vi "Main.vi"() -> ()   [LabVIEW 2021]
doc: "The myRIO Project template acquires acceleration data from the onboard accelerometer and displays the changes of acceleration values in a waveform chart."
uses:
  <vilib>/Platform/TimedLoop/XDataNode/timing_clust.ctl
  <vilib>/Platform/TimedLoop/XDataNode/nitl_modes.ctl
  <vilib>/Platform/TimedLoop/XDataNode/wakeup.ctl
  <vilib>/myRIO/Instrument Drivers/Onboard IO/I2C/typedefs/I2C User Configuration.ctl
  <vilib>/myRIO/Instrument Drivers/Onboard IO/I2C/typedefs/I2C Transfer Rate.ctl
  <vilib>/myRIO/Instrument Drivers/Onboard IO/I2C/typedefs/I2C Reference.ctl
  <vilib>/myRIO/Common/Instrument Driver Framework/Utilities/typedefs/myRIO Generic Hardware Reference.ctl
  <vilib>/myRIO/Common/Instrument Driver Framework/Utilities/typedefs/Hardware Version Enum.ctl
  <vilib>/myRIO/Common/Instrument Driver Framework/Utilities/typedefs/myRIO v1.0 Reference.ctl
  <vilib>/myRIO/Common/Instrument Driver Framework/Utilities/typedefs/Generic FPGA Reference.ctl
  <vilib>/myRIO/Common/Instrument Driver Framework/myRIO v1.0/I2C/typedefs/I2C Channels Enum.ctl
  <vilib>/myRIO/Instrument Drivers/Onboard IO/I2C/typedefs/I2C Configuration.ctl
  <vilib>/userDefined/High Color/nirio_resource_hc.ctl
  <vilib>/myRIO/Instrument Drivers/Onboard IO/UART/typedef/VISA Configuration.ctl
  <vilib>/myRIO/Instrument Drivers/Onboard IO/DIO/typedefs/DIO Reference.ctl
  <vilib>/myRIO/Common/Instrument Driver Framework/myRIO v1.0/DIO/typedefs/DIO Channels List.ctl
  <vilib>/myRIO/Common/Instrument Driver Framework/myRIO v1.0/DIO/typedefs/DIO Channels Enum.ctl
  <vilib>/myRIO/Instrument Drivers/Onboard IO/PWM/typedefs/PWM Reference.ctl
  <vilib>/myRIO/Common/Instrument Driver Framework/myRIO v1.0/PWM/typedefs/PWM Channels Enum.ctl
  <vilib>/myRIO/Instrument Drivers/Onboard IO/PWM/typedefs/PWM Configuration.ctl
  <vilib>/myRIO/Common/Instrument Driver Framework/Utilities/vis/Is FPGA Ref Available.vi
  <vilib>/myRIO/Common/Instrument Driver Framework/myRIO v1.0/I2C/vis/myRIO v1.1 Open I2C.vi
  <vilib>/myRIO/Instrument Drivers/Onboard IO/I2C/vis/Configure.vi
  <vilib>/myRIO/Instrument Drivers/Onboard IO/I2C/vis/Write.vi
  <vilib>/myRIO/Instrument Drivers/Onboard IO/I2C/vis/Read.vi
  5875c5f5-a436-469e-884c-53e7f58b3f13.vi
  <vilib>/myRIO/Common/Instrument Driver Framework/myRIO v1.0/DIO/vis/myRIO v1.1 Open DIO.vi
  <vilib>/myRIO/Instrument Drivers/Onboard IO/DIO/vis/Write.vi
  6fa42901-1153-49b1-957e-1088346b90ec.vi
  <vilib>/myRIO/Common/Instrument Driver Framework/myRIO v1.0/PWM/vis/myRIO v1.1 Open PWM.vi
  <vilib>/myRIO/Instrument Drivers/Onboard IO/PWM/vis/Set Duty Cycle and Frequency.vi
  <vilib>/myRIO/Instrument Drivers/Onboard IO/I2C/vis/Write Read.vi
  <vilib>/myRIO/Common/Instrument Driver Framework/Utilities/vis/Validate Channels.vi
  <vilib>/myRIO/Common/Instrument Driver Framework/myRIO v1.0/I2C/vis/myRIO v1.0 Reserve I2C.vi
  <vilib>/myRIO/Common/Instrument Driver Framework/myRIO v1.0/DIO/vis/myRIO v1.0 Reserve DIO.vi
  <vilib>/myRIO/Common/Instrument Driver Framework/myRIO v1.0/PWM/vis/myRIO v1.0 Reserve PWM.vi
  <vilib>/myRIO/Common/Instrument Driver Framework/myRIO v1.0/I2C/vis/myRIO v1.0 Build MUX Configuration I2C.vi
  <vilib>/myRIO/Common/Instrument Driver Framework/myRIO v1.0/Resource Manager/vis/myRIO v1.0 Reserve Channel List.vi
  <vilib>/myRIO/Common/Instrument Driver Framework/myRIO v1.0/DIO/vis/myRIO v1.0 Build MUX Configuration DIO.vi
  <vilib>/myRIO/Common/Instrument Driver Framework/myRIO v1.0/PWM/vis/myRIO v1.0 Build MUX Configuration PWM.vi
  <vilib>/myRIO/Common/Instrument Driver Framework/myRIO v1.0/Resource Manager/vis/myRIO v1.0 Create Configuration List.vi
  <vilib>/myRIO/Common/Instrument Driver Framework/myRIO v1.0/Resource Manager/vis/myRIO v1.0 Reserve Channel.vi
  <vilib>/myRIO/Common/Instrument Driver Framework/myRIO v1.0/Resource Manager/vis/myRIO v1.0 Unreserve Channel.vi
  <vilib>/myRIO/Common/Instrument Driver Framework/myRIO v1.0/Resource Manager/vis/myRIO v1.0 Build Mutex Name.vi
  <vilib>/Utility/VariantDataType/GetNumericInfo.vi
  <vilib>/Utility/error.llb/Error Cluster From Error Code.vi
  <vilib>/myRIO/Common/Instrument Driver Framework/myRIO v1.0/myRIO v1.1 Open.vi
  <vilib>/myRIO/Common/Instrument Driver Framework/Utilities/vis/IO Manager.vi
  <vilib>/myRIO/Common/Instrument Driver Framework/Utilities/vis/Configuration Manager.vi
  <vilib>/myRIO/Common/Instrument Driver Framework/myRIO v1.0/Resource Manager/vis/myRIO v1.0 Configure IO.vi
  <vilib>/myRIO/Common/Instrument Driver Framework/myRIO v1.0/myRIO v1.0 Close.vi
  <vilib>/myRIO/Common/Instrument Driver Framework/myRIO v1.0/I2C/vis/myRIO v1.0 Configure I2C.vi
  <vilib>/myRIO/Common/Instrument Driver Framework/myRIO v1.0/I2C/vis/myRIO v1.0 Write I2C.vi
  <vilib>/myRIO/Common/Instrument Driver Framework/myRIO v1.0/I2C/vis/myRIO v1.0 Read I2C.vi
  <vilib>/myRIO/Common/Instrument Driver Framework/myRIO v1.0/DIO/vis/myRIO v1.0 Write DIO.vi
  <vilib>/Instr/_visa.llb/VISA Configure Serial Port (Instr).vi
  <vilib>/myRIO/Common/Instrument Driver Framework/myRIO v1.0/PWM/vis/myRIO v1.0 Write PWM.vi
  <vilib>/myRIO/Express VI/Onboard IO/I2C/I2C Express VI.xnode
  <vilib>/myRIO/Instrument Drivers/Onboard IO/I2C/vis/myRIO I2C Open.xnode
  <vilib>/platform/TimedLoop/XDataNode/XDataNode.xnode
  <vilib>/myRIO/Express VI/Onboard IO/DO/DO Express VI.xnode
  <vilib>/myRIO/Instrument Drivers/Onboard IO/DIO/vis/myRIO DIO Open.xnode
  <vilib>/myRIO/Express VI/Onboard IO/UART/UART Express VI.xnode
  <vilib>/myRIO/Express VI/Onboard IO/PWM/PWM Express VI.xnode
  <vilib>/myRIO/Instrument Drivers/Onboard IO/PWM/vis/myRIO PWM Open.xnode
  <vilib>/myRIO/Instrument Drivers/Onboard IO/I2C/I2C.lvlib
  <vilib>/Platform/TimedLoop/XDataNode/XDNodeRunTimeDep.lvlib
  <vilib>/myRIO/Instrument Drivers/Onboard IO/UART/UART.lvlib
  <vilib>/myRIO/Instrument Drivers/Onboard IO/DIO/DIO.lvlib
  <vilib>/myRIO/Instrument Drivers/Onboard IO/PWM/PWM.lvlib
panel:
  in  "Set Prox.\nAlert [in]":i32=5
  out "Distance to Tree [in]":dbl(slide) scale=6.0..60.0
  out "Thermometer [C]":dbl(slide) scale=0.0..30.0
  in  "Set Low Temp\nAlert [Celsius]":dbl=-1.0 format="%#_13g"
  out "Error":errorcluster
  out "# of Tree Alerts":i16
  out "# of Cold\nAlerts":i16
  out "MAXSONAR out":string
  out "Temperature [Celsius]":dbl
  out "Tree Proximity [in]":i32
  out "XY Graph":cluster{i32[], i32[]}[](graph)
  in  "stop":bool
  in  "Reset To Cabin":bool
  out "CMPS2 Bytes Read":u8[](array[numeric])
  out "X Y Gauss":dbl[](array[numeric])
  out "CMPS2 Status Register":bool[](array[boolean])
  out "ACL INT SOURCE":bool[](array[boolean])
  out "ACL Bytes Read":u8[](array[numeric])
  out "X ACL":i16 format="%.1f"
  out "Y ACL":i16 format="%.1f"
  out "Z ACL":i16 format="%.1f"
  out "Acceleration":i16
  out "Walking":bool
  out "Compass Case":u32
  out "Compass\nHeading":string="E"
  # "CABIN"
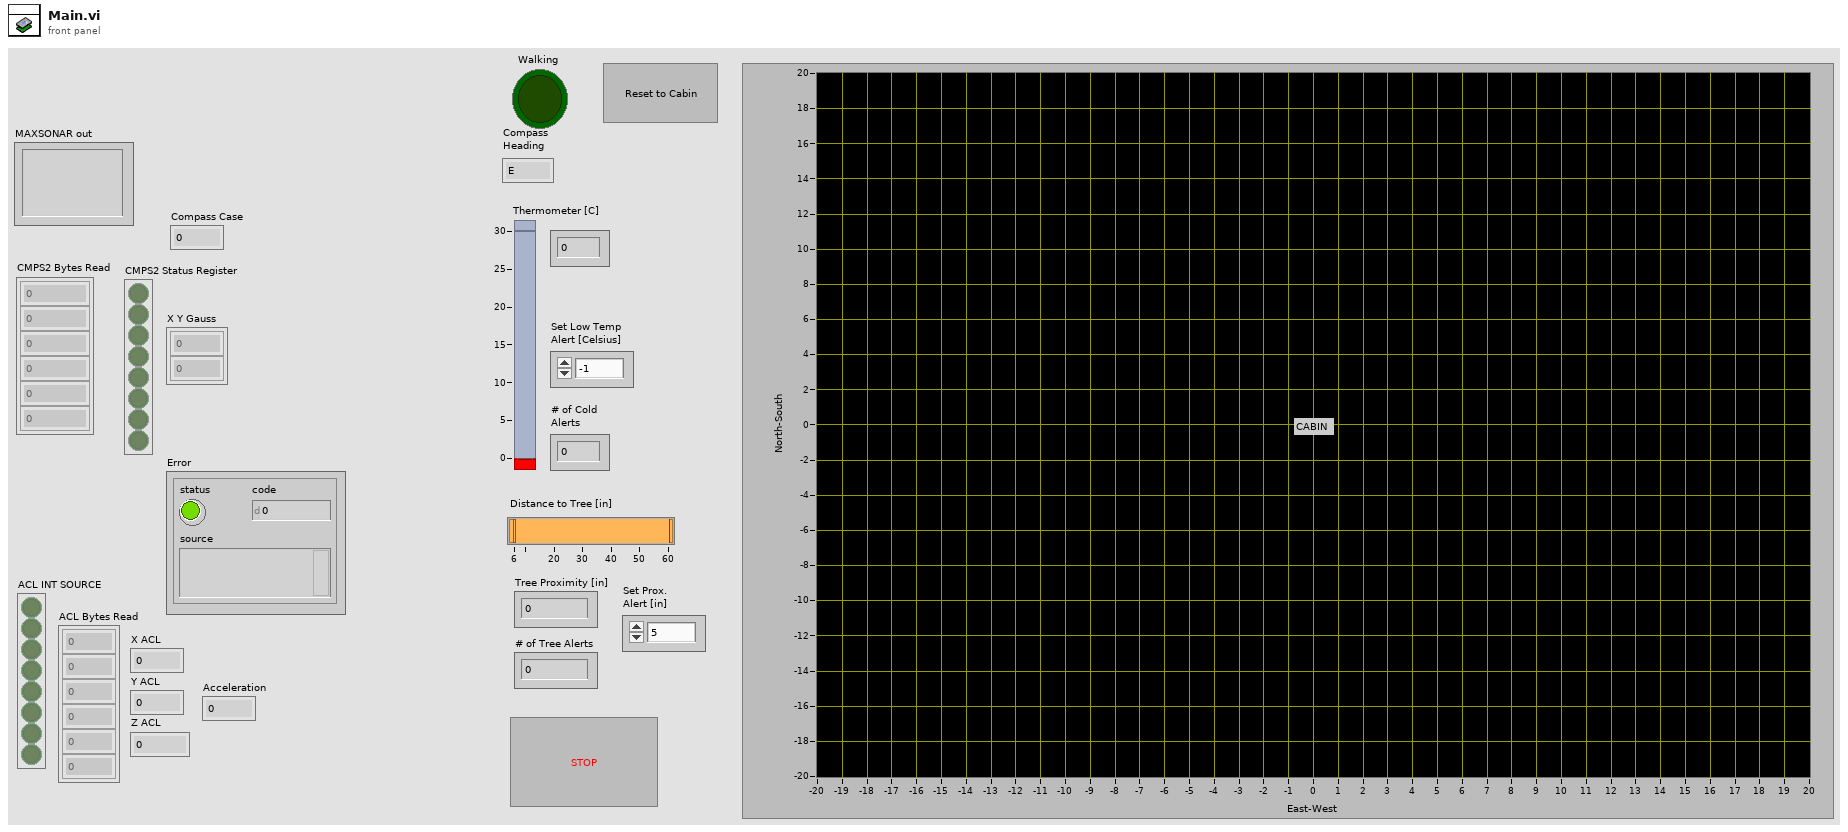
[diagram p1: front panel]
types:
  T1 = typedef "I2C.lvlib/I2C Reference.ctl" = cluster{"myRIO Reference":T2, "I2C Channels Enum":T6, "I2C Configuration":T7}
  T2 = typedef "myRIO Generic Hardware Reference.ctl" = cluster{"myRIO Model":T3, "myRIO Hardware Reference":T4}
  T3 = typedef "Hardware Version Enum.ctl" = enum16{"Unknown", "myRIO-1900", "myRIO-1950", "roboRIO", "NI ELVIS RIO CM", "ELVIS III"}
  T4 = typedef "myRIO v1.0 Reference.ctl" = cluster{"Generic FPGA Reference":T5, "Allow multiple opens":bool}
  T5 = typedef "Generic FPGA Reference.ctl" = refnum<k20>
  T6 = typedef "I2C Channels Enum.ctl" = enum16{"Not Connected", "A/I2C", "B/I2C", "I2C/I2C"}
  T7 = typedef "I2C.lvlib/I2C Configuration.ctl" = cluster{"I2C Transfer Rate":T8}
  T8 = typedef "I2C.lvlib/I2C Transfer Rate.ctl" = enum16{"Standard mode (100 kbps)", "Fast mode (400 kbps)"}
  T9 = typedef "I2C.lvlib/I2C User Configuration.ctl" = cluster{"I2C Transfer Rate":T8}
  T10 = typedef "nirio_resource_hc.ctl" = tag
  T11 = typedef "XDNodeRunTimeDep.lvlib/timing_clust.ctl" = cluster{"Expected End [f-1]":u64, "Actual End [f-1]":u64, "Finished Late? [f-1]":bool, "Expected End [i-1]":u64, "Actual End [i-1]":u64, "Finished Late? [i-1]":bool, "Expected Start [i]":u64, "Actual Start [i]":u64, "Expected Start [f]":u64, "Actual Start [f]":u64, "Source Name":string, "Structure Name":string, "Period":i64, "Deadline":i64, "Offset":i64, "Start":i64, "Priority":i32, "Timeout":i32, "Mode":T12, "Wakeup Reason":T13, "Error":errorcluster, "Source Type":string, "Secondary Source Type":string, "Global End Time":u64, "Global Start Time":u64, "Frame Duration":u64, "Iteration Duration":u64, "Assigned CPU":i32, "I/O Scan Engine Mode":u32}
  T12 = typedef "XDNodeRunTimeDep.lvlib/nitl_modes.ctl" = enum32{"No Change", "Process missed periods, maintain original phase", "Discard missed periods, maintain original phase", "Process missed periods, ignore original phase", "Discard missed periods, ignore original phase"}
  T13 = typedef "XDNodeRunTimeDep.lvlib/wakeup.ctl" = enum32{"Normal", "Aborted", "Asynchronous wakeup", "Timing source error", "Timed loop error", "Timeout"}
  T14 = typedef "PWM.lvlib/PWM Reference.ctl" = cluster{"myRIO Reference":T2, "PWM Channels Enum":T15, "PWM Configuration":T16}
  T15 = typedef "PWM Channels Enum.ctl" = enum16{"Not Connected", "C/PWM0", "C/PWM1", "A/PWM0", "A/PWM1", "A/PWM2", "A/PWM3", "A/PWM4", "A/PWM5", "A/PWM6", "A/PWM7", "A/PWM8", "A/PWM9", "A/PWM10", "A/PWM11", "A/PWM12", "A/PWM13", "A/PWM14", "A/PWM15", "A/PWM16", "A/PWM17", "A/PWM18", "A/PWM19", "B/PWM0", "B/PWM1", "B/PWM2", "B/PWM3", "B/PWM4", "B/PWM5", "B/PWM6", "B/PWM7", "B/PWM8", "B/PWM9", "B/PWM10", "B/PWM11", "B/PWM12", "B/PWM13", "B/PWM14", "B/PWM15", "B/PWM16", "B/PWM17", "B/PWM18", "B/PWM19", "PWM/PWM0", "PWM/PWM1", "PWM/PWM2", "PWM/PWM3", "PWM/PWM4", "PWM/PWM5", "PWM/PWM6", "PWM/PWM7", "PWM/PWM8", "PWM/PWM9"}
  T16 = typedef "PWM.lvlib/PWM Configuration.ctl" = cluster{"Frequency":dbl, "Duty Cycle":dbl}
  T17 = typedef "DIO.lvlib/DIO Reference.ctl" = cluster{"myRIO Reference":T2, "DIO Channels List":T18}
  T18 = typedef "DIO Channels List.ctl" = T19[]
  T19 = typedef "DIO Channels Enum.ctl" = enum16{"Not Connected", "C/DIO0", "C/DIO1", "C/DIO2", "C/DIO3", "C/DIO4", "C/DIO5", "C/DIO6", "C/DIO7", "A/DIO0", "A/DIO1", "A/DIO2", "A/DIO3", "A/DIO4", "A/DIO5", "A/DIO6", "A/DIO7", "A/DIO8", "A/DIO9", "A/DIO10", "A/DIO11", "A/DIO12", "A/DIO13", "A/DIO14", "A/DIO15", "A/DIO16", "A/DIO17", "A/DIO18", "A/DIO19", "B/DIO0", "B/DIO1", "B/DIO2", "B/DIO3", "B/DIO4", "B/DIO5", "B/DIO6", "B/DIO7", "B/DIO8", "B/DIO9", "B/DIO10", "B/DIO11", "B/DIO12", "B/DIO13", "B/DIO14", "B/DIO15", "B/DIO16", "B/DIO17", "B/DIO18", "B/DIO19", "LED0", "LED1", "LED2", "LED3", "Button0", "DIO/DIO0", "DIO/DIO1", "DIO/DIO2", "DIO/DIO3", "DIO/DIO4", "DIO/DIO5", "DIO/DIO6", "DIO/DIO7", "DIO/DIO8", "DIO/DIO9", "SPI/CS0", "SPI/CS1", "SPI/CS2", "SPI/CS3", "LED RADIO (Green)", "LED RADIO (Red)", "LED COMM (Green)", "LED COMM (Red)", "LED MODE (Green)", "LED MODE (Red)"}
  T20 = typedef "UART.lvlib/VISA Configuration.ctl" = cluster{"baud rate (9600)":u32, "data bits (8)":u16, "parity (0:none)":enum16{"None", "Odd", "Even", "Mark", "Space"}, "stop bits (10: 1 bit)":u16, "flow control (0:none)":u16, "termination char\n(0xA = '\\n' = LF) ":u8, "Enable Termination\nChar (T)":bool, "timeout (10sec)":u32}
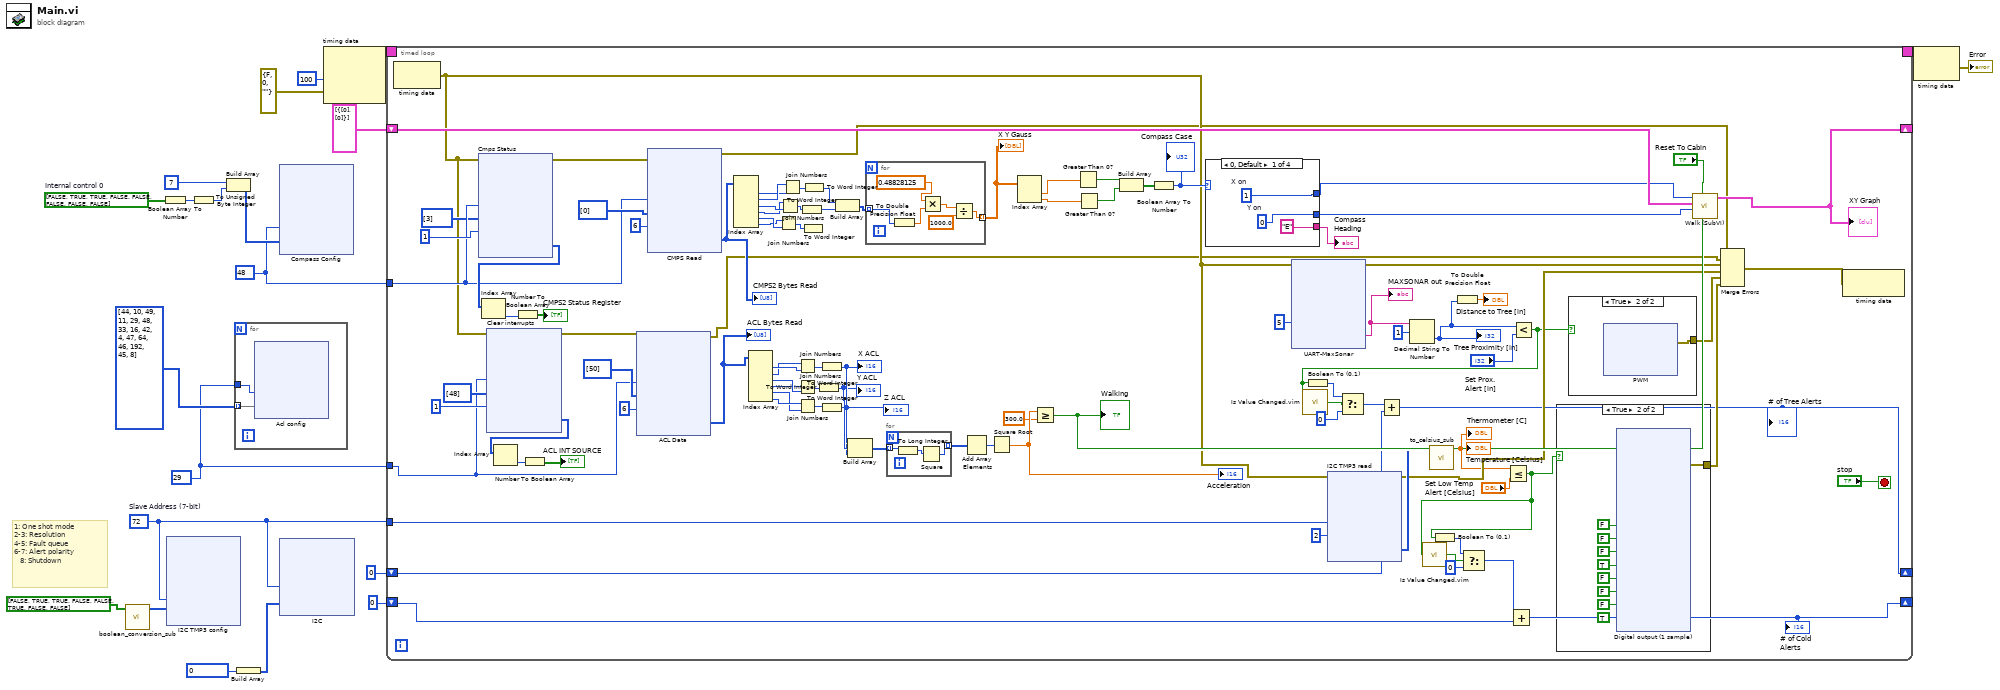
[diagram p0: block diagram]
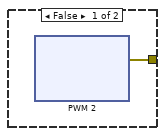
[diagram p2: hidden frame]
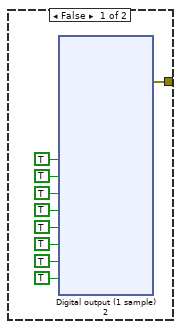
[diagram p3: hidden frame]
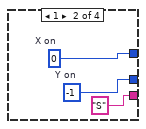
[diagram p4: hidden frame]
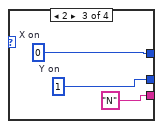
[diagram p5: hidden frame]
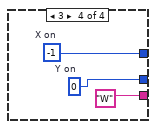
[diagram p6: hidden frame]
diagram:
  w8 = u8 29 ("Slave Address (7-bit)")
  w11 = u8 48
  w12 = bool[] [FALSE, TRUE, TRUE, FALSE, FALSE, FALSE, FALSE, FALSE]  # Internal control 0
  w7 = u8 72  # Slave Address (7-bit)
  # "1: One shot mode\n2-3: Resolution \n4-5: Fault queue\n6-7: Alert polarity\n   8: Shutdown"
  n1 = call "boolean_conversion_sub.vi"("Array in"=bool[] [FALSE, TRUE, TRUE, FALSE, FALSE, TRUE, FALSE, FALSE]) -> ("Array out"=w20:u8[])  [unwired: 10 in]
  n2 = Boolean Array To Number(Boolean array=w12) -> (number=w16:u32)
  n3 = xnode "I2C TMP3 config"("Slave Address (7-bit)"=w7, "Bytes to Write"=w20) -> ()  [unwired: 1 in, 1 out]
  n4 = To Unsigned Byte Integer(number=w16) -> (unsigned 8bit integer=w14:u8)
  n5 = Build Array(u8 7, w14) -> (w15:u8[])
  n6 = for {
    tunnel: w8 -> [w23]
    tunnel: u8[][] [[44, 10], [49, 11], [29, 48], [33, 16], [42, 4], [47, 64], [46, 192], [45, 8]] -> [w22] mode=indexing
    n7 = xnode "Acl config"("Slave Address (7-bit)"=w23, "Bytes to Write"=w22) -> ()  [unwired: 1 in, 1 out]
  }
  n8 = Build Array(u8 0) -> (w5:u8[])
  n9 = xnode "Compass Config"("Slave Address (7-bit)"=w11, "Bytes to Write"=w15) -> ()  [unwired: 1 in, 1 out]
  n10 = xnode "I2C"("Slave Address (7-bit)"=w7, "Bytes to Write"=w5) -> ()  [unwired: 1 in, 1 out]
  n11 = node-c288(i64 100 ("Period"), errorcluster {"status"=FALSE, "code"=0, "source"=""} ("Error")) -> (w19:T11)  [unwired: 1 in]
  n12 = timed-loop {
    timing: w19 -> [_]
    timing-out: [_] -> w18
    shift-right: [w97] -> _
    shift-left: cluster{"X Cord":i32[], "Y Cord":i32[]}[] [{"X Cord"=[0], "Y Cord"=[0]}] -> [w109]
    tunnel: w11 -> [w137]
    tunnel: w8 -> [w112]
    tunnel: w7 -> [w87]
    shift-right: [w84] -> _
    shift-left: i16 0 -> [w85]
    shift-right: [w82] -> _
    shift-left: i16 0 -> [w83]
    stop <- "stop" stop-if-true
    n13 = node-c288() -> (w68:errorcluster)  [unwired: 1 in]
    n14 = xnode "Cmps Status"("Slave Address (7-bit)"=w137, "Bytes to Write"=u8[] [3], "Byte Count"=u32 1, "error in (no error)"=w68) -> ("Bytes Read"=w152:u8[], "error out"=w70:errorcluster)
    n15 = Index Array(array=w152) -> (element=w150:u8)  [unwired: 1 in]
    n16 = xnode "Clear interrupts"("Slave Address (7-bit)"=w112, "Bytes to Write"=u8[] [48], "Byte Count"=u32 1, "error in (no error)"=w68) -> ("Bytes Read"=w133:u8[], "error out"=w69:errorcluster)
    n17 = Index Array(array=w133) -> (element=w132:u8)  [unwired: 1 in]
    n18 = Number To Boolean Array(number=w150) -> (Boolean array=→"CMPS2 Status Register":bool[])
    n19 = Number To Boolean Array(number=w132) -> (Boolean array=→"ACL INT SOURCE":bool[])
    n20 = xnode "ACL Data"("Slave Address (7-bit)"=w112, "Bytes to Write"=u8[] [50], "Byte Count"=u32 6, "error in (no error)"=w69) -> ("Bytes Read"=w128:u8[], "error out"=w66:errorcluster)
    "ACL Bytes Read" <- w128
    n21 = xnode "CMPS Read"("Slave Address (7-bit)"=w137, "Bytes to Write"=u8[] [0], "Byte Count"=u32 6, "error in (no error)"=w70) -> ("Bytes Read"=w156:u8[], "error out"=w67:errorcluster)
    "CMPS2 Bytes Read" <- w156
    n22 = Index Array(array=w156) -> (element #1=w147:u8, element #2=w148:u8, element #3=w146:u8, element #4=w145:u8, element #5=w144:u8, element #6=w143:u8)  [unwired: 6 in]
    n23 = Index Array(array=w128) -> (element #1=w127:u8, element #2=w126:u8, element #3=w125:u8, element #4=w124:u8, element #5=w122:u8, element #6=w123:u8)  [unwired: 6 in]
    n24 = Join Numbers(hi=w143, lo=w144) -> ((hi.lo)=w138:u16)
    n25 = Join Numbers(hi=w145, lo=w146) -> ((hi.lo)=w140:u16)
    n26 = Join Numbers(hi=w148, lo=w147) -> ((hi.lo)=w142:u16)
    n27 = Join Numbers(hi=w126, lo=w127) -> ((hi.lo)=w120:u16)
    n28 = Join Numbers(hi=w124, lo=w125) -> ((hi.lo)=w121:u16)
    n29 = Join Numbers(hi=w123, lo=w122) -> ((hi.lo)=w119:u16)
    n30 = To Word Integer(number=w140) -> (16bit integer=w139:i16)
    n31 = To Word Integer(number=w138) -> ()  [unwired: 1 out]
    n32 = To Word Integer(number=w142) -> (16bit integer=w141:i16)
    n33 = To Word Integer(number=w121) -> (16bit integer=w117:i16)
    "Y ACL" <- w117
    n34 = To Word Integer(number=w120) -> (16bit integer=w118:i16)
    "X ACL" <- w118
    n35 = To Word Integer(number=w119) -> (16bit integer=w116:i16)
    "Z ACL" <- w116
    n36 = Build Array(w141, w139) -> (w155:i16[])
    n37 = Build Array(w118, w117, w116) -> (w115:i16[])
    n38 = for {
      tunnel: w155 -> [w487] mode=indexing
      tunnel: [w485] -> w107 mode=indexing
      n39 = To Double Precision Float(number=w487) -> (double precision float=w486:dbl)
      n40 = Multiply(x=0.48828125, y=w486) -> (x*y=w484:dbl)
      n41 = Divide(x=w484, y=1000.0) -> (x/y=w485:dbl)
    }
    "X Y Gauss" <- w107
    n42 = for {
      tunnel: w115 -> [w400] mode=indexing
      tunnel: [w402] -> w114 mode=indexing
      n43 = To Long Integer(number=w400) -> (32bit integer=w401:i32)
      n44 = Square(x=w401) -> (x^2=w402:i32)
    }
    n45 = Add Array Elements(numeric array=w114) -> (sum=w113:i32)
    n46 = Square Root(x=w113) -> (sqrt(x)=w111:dbl)
    "Acceleration" <- w111
    n47 = Index Array(array=w107) -> (element #1=w106:dbl, element #2=w105:dbl)  [unwired: 2 in]
    n48 = Greater Or Equal?(x=w111, y=300.0) -> (x >= y?=w108:bool)
    "Walking" <- w108
    n49 = Greater Than 0?(x=w106) -> (x > 0?=w103:bool)
    n50 = Greater Than 0?(x=w105) -> (x > 0?=w104:bool)
    n51 = Build Array(w103, w104) -> (w102:bool[])
    n52 = Boolean Array To Number(Boolean array=w102) -> (number=w101:u32)
    "Compass Case" <- w101
    n53 = case shown="0, Default" w101 {
      tunnel: [w389 w392 w395 w399] -> w100
      tunnel: [w390 w393 w396 w398] -> w99
      tunnel: ["E" "S" "N" "W"] -> w98
      frame 0, Default {
        w390 = 1  # X on
        w389 = 0  # Y on
      }
      frame 1 {
        w393 = 0  # X on
        w392 = -1  # Y on
      }
      frame 2 {
        w396 = 0  # X on
        w395 = 1  # Y on
      }
      frame 3 {
        w398 = -1  # X on
        w399 = 0  # Y on
      }
    }
    "Compass\nHeading" <- w98
    n54 = xnode "UART-MaxSonar"("Character Count"=u32 5, "error in (no error)"=w68) -> ("Characters Read"=w92:string, "error out"=w94:errorcluster)
    "MAXSONAR out" <- w92
    n55 = xnode "I2C TMP3 read"("Slave Address (7-bit)"=w87, "Byte Count"=u32 2, "error in (no error)"=w68) -> ("Bytes Read"=w96:u8[], "error out"=w95:errorcluster)
    n56 = Decimal String To Number(string=w92, offset=1) -> (number=w63:i32)  [unwired: 1 in, 1 out]
    "Tree Proximity [in]" <- w63
    n57 = call "to_celsius_sub.vi"("Bytes Read"=w96) -> ("Numeric"=w64:dbl)  [unwired: 10 in]
    "Temperature [Celsius]" <- w64
    "Thermometer [C]" <- w64
    n58 = To Double Precision Float(number=w63) -> (double precision float=→"Distance to Tree [in]":dbl)
    n59 = Less Or Equal?(x=w64, y="Set Low Temp\nAlert [Celsius]") -> (x <= y?=w71:bool)
    n60 = call "Is Value Changed.vim"("value"=w71) -> ("changed or first call?"=w81:bool)
    n61 = Boolean To (0,1)(Boolean=w71) -> (0, 1=w80:i16)
    n62 = Select(t=w80, s=w81, f=i16 0) -> (s? t:f=w78:i16)
    n63 = Add(x=w78, y=w85) -> (x+y=w84:i16)
    "# of Cold\nAlerts" <- w84
    n64 = Less?(x=w63, y="Set Prox.\nAlert [in]") -> (x < y?=w76:bool)
    n65 = call "Is Value Changed.vim"("value"=w76) -> ("changed or first call?"=w77:bool)
    n66 = Boolean To (0,1)(Boolean=w76) -> (0, 1=w75:i16)
    n67 = Select(t=w75, s=w77, f=i16 0) -> (s? t:f=w73:i16)
    n68 = Add(x=w73, y=w83) -> (x+y=w82:i16)
    "# of Tree Alerts" <- w82
    n69 = case shown="True" w71 {
      tunnel: [w231 w282] -> w88
      frame False {
        n70 = xnode "Digital output (1 sample) 2"("pin a (B/DIO0 (Pin 11))"=TRUE, "pin b (B/DIO1 (Pin 13))"=TRUE, "pin c (B/DIO2 (Pin 15))"=TRUE, "pin d (B/DIO3 (Pin 17))"=TRUE, "pin e (B/DIO4 (Pin 19))"=TRUE, "pin f (B/DIO5 (Pin 21))"=TRUE, "pin g (B/DIO6 (Pin 23))"=TRUE, "pin dp (B/DIO7 (Pin 25))"=TRUE) -> ("error out"=w231:errorcluster)  [unwired: 1 in]
      }
      frame True {
        n71 = xnode "Digital output (1 sample)"("pin a (B/DIO0 (Pin 11))"=FALSE, "pin b (B/DIO1 (Pin 13))"=FALSE, "pin c (B/DIO2 (Pin 15))"=FALSE, "pin d (B/DIO3 (Pin 17))"=TRUE, "pin e (B/DIO4 (Pin 19))"=FALSE, "pin f (B/DIO5 (Pin 21))"=FALSE, "pin g (B/DIO6 (Pin 23))"=FALSE, "pin dp (B/DIO7 (Pin 25))"=TRUE) -> ("error out"=w282:errorcluster)  [unwired: 1 in]
      }
    }
    n72 = case shown="True" w76 {
      tunnel: [w159 w195] -> w89
      frame False {
        n73 = xnode "PWM 2"() -> ("error out"=w159:errorcluster)  [unwired: 1 in]
      }
      frame True {
        n74 = xnode "PWM"() -> ("error out"=w195:errorcluster)  [unwired: 1 in]
      }
    }
    n75 = call "Walk (SubVI).vi"("Boolean"=w108, "Reset To Cabin"="Reset To Cabin", "Y"=w100, "Array in"=w109, "X"=w99) -> ("Array out"=w97:cluster{"Y":i32[], "\nX":i32[]}[])  [unwired: 6 in]
    "XY Graph" <- w97
    n76 = Merge Errors(w67, w66, w94, w95, w89, w88) -> (w65:errorcluster)
    n77 = node-c288(w65) -> ()  [unwired: 1 out]
  }
  n78 = node-c288(w18) -> (→"Error":errorcluster)
